vi "MPB Signal Writes.vi"() -> (3 "TX Signals":string[](array[string])=["AEthernet.Powertrain.TCU.RX_PDUs.MPB_STS_1.IMPB_CntctSts1", "AEthernet.Powertrain.TCU.RX_PDUs.MPB_STS_1.IMPB_CntctSts2", "AEthernet.Powertrain.TCU.RX_PDUs.MPB_STS_1.IMPB_CntctSts3", "AEthernet.Powertrain.TCU.RX_PDUs.MPB_STS_1.IMPB_CntctSts4", "AEthernet.Powertrain.TCU.RX_PDUs.MPB_STS_1.IMPB_CntctSts5", "AEthernet.Powertrain.TCU.RX_PDUs.MPB_STS_1.IMPB_CntctSts6", "AEthernet.Powertrain.TCU.RX_PDUs.MPB_STS_1.IMPB_CntctSts7", "AEthernet.Powertrain.TCU.RX_PDUs.MPB_STS_1.IMPB_RlySts1", "AEthernet.Powertrain.TCU.RX_PDUs.MPB_STS_1.IMPB_RlySts2", "AEthernet.Powertrain.TCU.RX_PDUs.MPB_STS_1.IMPB_BattCurrDAB1", "AEthernet.Powertrain.TCU.RX_PDUs.MPB_STS_1.IMPB_BattCurrDAB2", "AEthernet.Powertrain.TCU.RX_PDUs.MPB_STS_1.IMPB_BattVoltgHiRes", "AEthernet.Powertrain.TCU.RX_PDUs.MPB_STS_1.IMPB_DCbusVoltg", "AEthernet.Powertrain.TCU.RX_PDUs.MPB_STS_1.IMPB_BattPortPower", "AEthernet.Powertrain.TCU.RX_PDUs.MPB_STS_1.IMPB_InletDCportVoltgHiRes", "AEthernet.Powertrain.TCU.RX_PDUs.MPB_INLET_1.IMPB_DCbusVoltgLowrHalf", "AEthernet.Powertrain.TCU.RX_PDUs.MPB_STS_1.IMPB_BattPortVoltgLowRes", "AEthernet.Powertrain.TCU.RX_PDUs.MPB_HAPS.IMPB_HAPSVoltgIn", "AEthernet.Powertrain.TCU.RX_PDUs.MPB_HwFlt.IMPB_HwFltCode", "AEthernet.Powertrain.TCU.RX_PDUs.MPB_STS_1.IMPB_BattPortNegFuseLowRes", "AEthernet.Powertrain.TCU.RX_PDUs.MPB_STS_1.IMPB_BattPortPosFuseLowRes", "AEthernet.Powertrain.TCU.RX_PDUs.MPB_HwFlt.IMPB_HwFltFlag", "AEthernet.Powertrain.TCU.RX_PDUs.MPB_ACCURR.IMPB_ACCurr1", "AEthernet.Powertrain.TCU.RX_PDUs.MPB_ACCURR.IMPB_ACCurr2", "AEthernet.Powertrain.TCU.RX_PDUs.MPB_ACCURR.IMPB_ACCurr3", "AEthernet.Powertrain.TCU.RX_PDUs.MPB_ACCURR.IMPB_ACCurr4", "AEthernet.Powertrain.TCU.RX_PDUs.MPB_HAPS.IMPB_HAPSCurr", "AEthernet.Powertrain.TCU.RX_PDUs.MPB_HAPS.IMPB_HAPSVoltgOut", "AEthernet.Powertrain.TCU.RX_PDUs.MPB_HAPS.IMPB_HAPSFltFlag", "AEthernet.Powertrain.TCU.RX_PDUs.MPB_HAPS.IMPB_HAPSFltCode"])   [LabVIEW 2020]
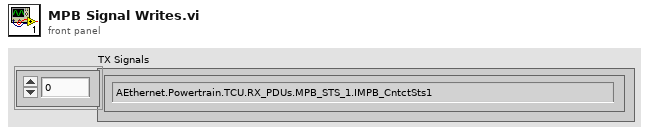
[diagram p1: front panel]
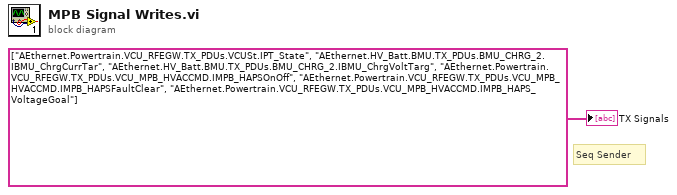
[diagram p0: block diagram]
diagram:
  # "Seq Sender"
  "TX Signals" <- string[] ["AEthernet.Powertrain.VCU_RFEGW.TX_PDUs.VCUSt.IPT_State", "AEthernet.HV_Batt.BMU.TX_PDUs.BMU_CHRG_2.IBMU_ChrgCurrTar", "AEthernet.HV_Batt.BMU.TX_PDUs.BMU_CHRG_2.IBMU_ChrgVoltTarg", "AEthernet.Powertrain.VCU_RFEGW.TX_PDUs.VCU_MPB_HVACCMD.IMPB_HAPSOnOff", "AEthernet.Powertrain.VCU_RFEGW.TX_PDUs.VCU_MPB_HVACCMD.IMPB_HAPSFaultClear", "AEthernet.Powertrain.VCU_RFEGW.TX_PDUs.VCU_MPB_HVACCMD.IMPB_HAPS_VoltageGoal"]
